vi "SetParam.vi"(8 "error in (no error)":errorcluster caption="entrée d'erreur (pas d'erreur)", 10 "make_sparse_uncorrelated":T1={"n_samples"=100, "n_features"=10, "random_state"=-1, "Returns"="X"} {"random_state" min=-1; "n_samples" min=1}, 11 "Sparse_Uncorrelated.lvclass":refnum<class "Sparse_Uncorrelated.lvclass">) -> (0 "error out":errorcluster caption="sortie d'erreur", 3 "Sparse_Uncorrelated.lvclass":refnum<class "Sparse_Uncorrelated.lvclass">)   [LabVIEW 2020, in "Sparse_Uncorrelated.lvclass"]
doc: "Set Parameters"
uses:
  Sparse_Uncorrelated.lvclass
  Sparse_Uncorrelated.lvclass/Sparse_Uncorrelated.ctl
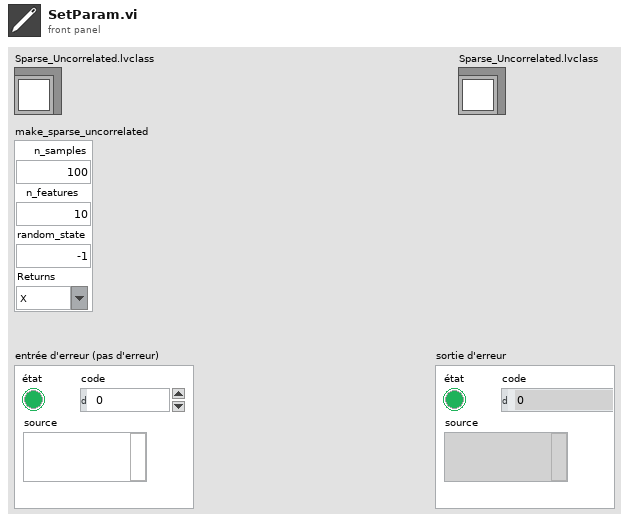
[diagram p1: front panel]
types:
  T1 = cluster{"n_samples":u32, "n_features":i32, "random_state":i32, "Returns":string}
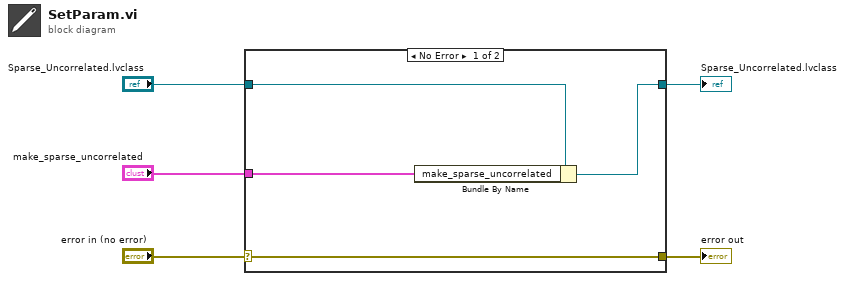
[diagram p0: block diagram]
diagram:
  n1 = case shown="No Error" "error in (no error)" {
    selector: "error in (no error)" -> [w9 w10]
    tunnel: [w9 w10] -> w4
    tunnel: [w7 w11] -> w2
    tunnel: "Sparse_Uncorrelated.lvclass" -> [w8 w11]
    tunnel: "make_sparse_uncorrelated" -> [w6 _]
    frame No Error {
      n2 = Bundle By Name(cluster=w8, "make_sparse_uncorrelated"=w6) -> (w7:refnum<class "Sparse_Uncorrelated.lvclass">)
    }
    frame Error {
    }
  }
  "error out" <- w4
  "Sparse_Uncorrelated.lvclass" <- w2
